vi "RGBA2Color.vi"(11 "RGBA":cluster{"R":sgl, "G":sgl, "B":sgl, "A":sgl}) -> (2 "Alpha":dbl=1.0, 3 "Color":u32(colorbox))   [LabVIEW 2014]
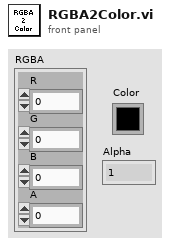
[diagram p1: front panel]
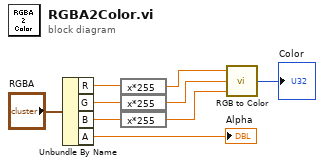
[diagram p0: block diagram]
diagram:
  n1 = Unbundle By Name("RGBA") -> ("R"=w8:sgl, "G"=w7:sgl, "B"=w6:sgl, "A"=→"Alpha":sgl)
  n2 = expression code="x*255"(w8) -> (w4:sgl)
  n3 = expression code="x*255"(w7) -> (w3:sgl)
  n4 = expression code="x*255"(w6) -> (w2:sgl)
  n5 = call <vilib>:"RGB to Color.vi"("B"=w2, "G"=w3, "R"=w4) -> ("Color"=→"Color":u32)
